vi "Combine two 1D arrays.vi"(1 "Array2":dbl[](array[numeric]), 2 "Array1":dbl[](array[numeric])) -> (0 "Combined array":dbl[][](array[numeric]))   [LabVIEW 2009, in "Varian Magnet.lvclass"]
uses:
  Varian Magnet.lvclass
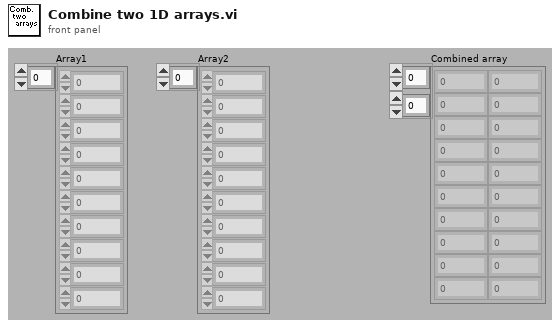
[diagram p1: front panel]
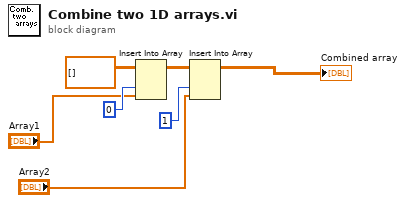
[diagram p0: block diagram]
diagram:
  n1 = Insert Into Array(array=dbl[][] [] ("appended array 2"), index (col)=0 ("index (row)"), new element="Array1") -> (w6:dbl[][])  [unwired: 1 in]
  n2 = Insert Into Array(array=w6, index (col)=1 ("disabled index (col)"), new element="Array2") -> (→"Combined array":dbl[][])  [unwired: 1 in]
